vi "String to Task.vi"(11 "Get_Val":string) -> (3 "Refnum out":refnum<k21>)   [LabVIEW 2021, in "NI DAQmx_wrapper.lvlib"]
uses:
  NI DAQmx_wrapper.lvlib
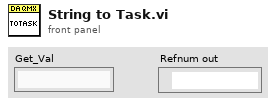
[diagram p1: front panel]
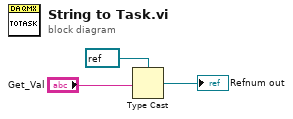
[diagram p0: block diagram]
diagram:
  n1 = Type Cast(type=refnum<k21> refnum ("task in"), x="Get_Val") -> (*(type *) &x=→"Refnum out":refnum<k21>)
